vi "New Mapped Lookup.vi"(8 "error in (no error)":errorcluster) -> (0 "error out":errorcluster, 3 "New Mapped Lookup":refnum<data-value>)   [LabVIEW 2019, in "LVCOOOP.lvlib" / "Lookup API.lvlib" / "Mapped Lookup.lvclass"]
uses:
  Mapped Lookup.lvclass
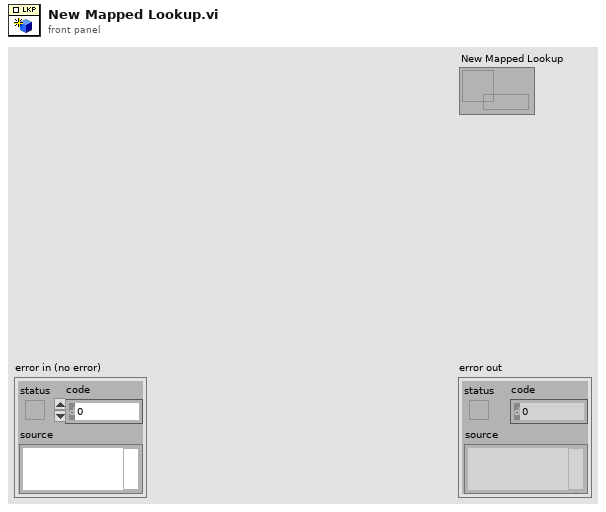
[diagram p1: front panel]
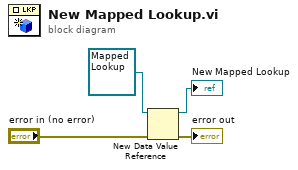
[diagram p0: block diagram]
diagram:
  n1 = New Data Value Reference(data value=refnum<class "Mapped Lookup.lvclass"> refnum ("Mapped Lookup in"), error in="error in (no error)") -> (data value reference=→"New Mapped Lookup":refnum<data-value>, error out=→"error out":errorcluster)
